vi "Get Adjacent.vi"(8 "Side":T1, 9 "Column In":i32, 10 "Row In":i32, 11 "Array In":u8[][](array[numeric])) -> (1 "Column Out":i32[](array[numeric]), 2 "Row Out":i32[](array[numeric]), 3 "Array":u8[](array[numeric]))   [LabVIEW 2019, in "Day 15.lvlib"]
uses:
  Day 15.lvlib
  Controls/Side.ctl
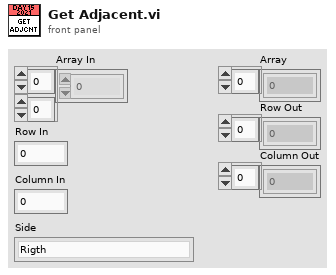
[diagram p1: front panel]
types:
  T1 = typedef "Day 15.lvlib/Side.ctl" = enum16{"Rigth", "Left", "Down", "Up", "Rigth Up", "Rigth Down", "Left Up", "Left Down"}
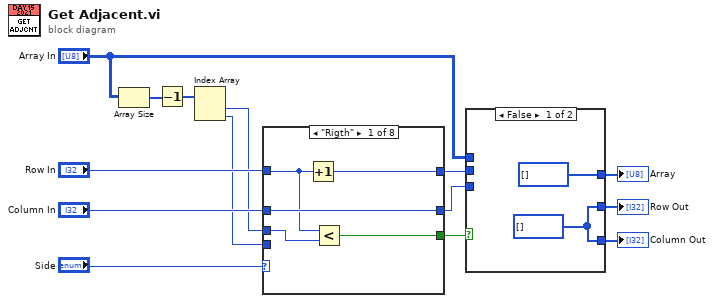
[diagram p0: block diagram]
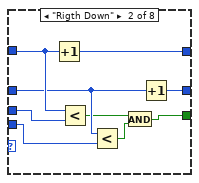
[diagram p2: hidden frame]
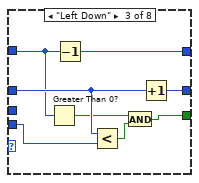
[diagram p3: hidden frame]
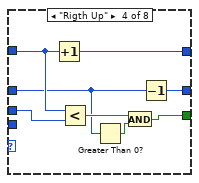
[diagram p4: hidden frame]
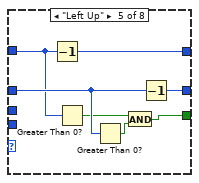
[diagram p5: hidden frame]
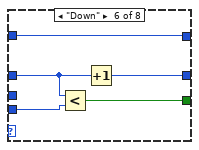
[diagram p6: hidden frame]
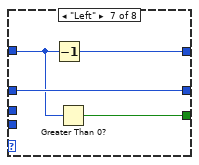
[diagram p7: hidden frame]
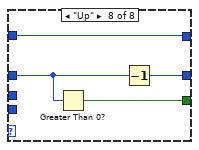
[diagram p8: hidden frame]
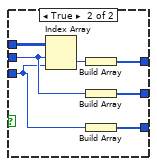
[diagram p9: hidden frame]
diagram:
  n1 = Array Size(array="Array In") -> (size(s)=w13:i32[])
  n2 = Decrement(x=w13) -> (x-1=w12:i32[])
  n3 = Index Array(array=w12) -> (element #1=w6:i32, element #2=w5:i32)  [unwired: 2 in]
  n4 = case shown="\"Rigth\"" "Side" {
    tunnel: "Row In" -> [w17 w27 w30 w43 w46 w56 w58 w64]
    tunnel: "Column In" -> [w19 w24 w35 w38 w49 w53 w60 w62]
    tunnel: [w19 w25 w36 w41 w51 w52 w60 w61] -> w7
    tunnel: [w18 w28 w31 w44 w47 w56 w59 w64] -> w8
    tunnel: w6 -> [w16 w26 _ w42 _ _ _ _]
    tunnel: w5 -> [_ w23 w34 _ _ w54 _ _]
    tunnel: [w15 w20 w32 w39 w50 w55 w57 w63] -> w4
    frame "Rigth" {
      n5 = Increment(x=w17) -> (x+1=w18:i32)
      n6 = Less?(x=w17, y=w16) -> (x < y?=w15:bool)
    }
    frame "Rigth Down" {
      n7 = Increment(x=w27) -> (x+1=w28:i32)
      n8 = Less?(x=w27, y=w26) -> (x < y?=w22:bool)
      n9 = Less?(x=w24, y=w23) -> (x < y?=w21:bool)
      n10 = And(x=w22, y=w21) -> (x .and. y?=w20:bool)
      n11 = Increment(x=w24) -> (x+1=w25:i32)
    }
    frame "Left Down" {
      n12 = Greater Than 0?(x=w30) -> (x > 0?=w29:bool)
      n13 = Decrement(x=w30) -> (x-1=w31:i32)
      n14 = Less?(x=w35, y=w34) -> (x < y?=w33:bool)
      n15 = And(x=w29, y=w33) -> (x .and. y?=w32:bool)
      n16 = Increment(x=w35) -> (x+1=w36:i32)
    }
    frame "Rigth Up" {
      n17 = Increment(x=w43) -> (x+1=w44:i32)
      n18 = Less?(x=w43, y=w42) -> (x < y?=w40:bool)
      n19 = Greater Than 0?(x=w38) -> (x > 0?=w37:bool)
      n20 = And(x=w40, y=w37) -> (x .and. y?=w39:bool)
      n21 = Decrement(x=w38) -> (x-1=w41:i32)
    }
    frame "Left Up" {
      n22 = Decrement(x=w46) -> (x-1=w47:i32)
      n23 = Greater Than 0?(x=w46) -> (x > 0?=w45:bool)
      n24 = Greater Than 0?(x=w49) -> (x > 0?=w48:bool)
      n25 = And(x=w45, y=w48) -> (x .and. y?=w50:bool)
      n26 = Decrement(x=w49) -> (x-1=w51:i32)
    }
    frame "Down" {
      n27 = Less?(x=w53, y=w54) -> (x < y?=w55:bool)
      n28 = Increment(x=w53) -> (x+1=w52:i32)
    }
    frame "Left" {
      n29 = Decrement(x=w58) -> (x-1=w59:i32)
      n30 = Greater Than 0?(x=w58) -> (x > 0?=w57:bool)
    }
    frame "Up" {
      n31 = Greater Than 0?(x=w62) -> (x > 0?=w63:bool)
      n32 = Decrement(x=w62) -> (x-1=w61:i32)
    }
  }
  n33 = case shown="False" w4 {
    tunnel: w8 -> [_ w70]
    tunnel: "Array In" -> [_ w73]
    tunnel: w7 -> [_ w69]
    tunnel: [u8[] [] w71] -> w14
    tunnel: [w65 w68] -> w2
    tunnel: [w65 w67] -> w3
    frame False {
      w65 = i32[] []
    }
    frame True {
      n34 = Index Array(array=w73, index (row)=w70, index (col)=w69) -> (element=w72:u8)
      n35 = Build Array(w72) -> (w71:u8[])
      n36 = Build Array(w70) -> (w68:i32[])
      n37 = Build Array(w69) -> (w67:i32[])
    }
  }
  "Array" <- w14
  "Row Out" <- w2
  "Column Out" <- w3
